vi "Intake Set.vi"() -> ()   [LabVIEW 2017]
uses:
  <vilib>/Rock Robotics/WPI/DriverStation/WPI_DriverStationRobotMode2.ctl
  Intake Control Type.ctl
  Intake Globals.vi
  Robot Global Data.vi
panel:
  out "error out 2":errorcluster
  out "error out":errorcluster
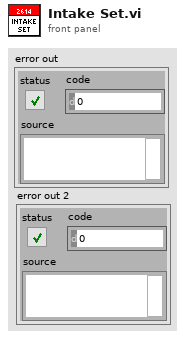
[diagram p1: front panel]
types:
  T1 = typedef "Intake Control Type.ctl" = enum16{"No Op", "In", "Out", "Test Mode", "Cube_In", "Cube_Out"}
  T2 = typedef "WPI_DriverStationRobotMode2.ctl" = enum16{"Autonomous Disabled", "Autonomous Enabled", "Teleop Disabled", "Teleop Enabled", "Disconnected", "Finish", "Test Disabled", "Test Enabled", "Emergency Stopped"}
  T3 = typedef "Intake Notifier.ctl" = cluster{"Intake Control Type":T1, "Step":i32, "In":bool, "Speed":dbl, "Out":bool, "Parameter 1":dbl, "Parameter 2":dbl, "Intake Notifier":refnum<notifier>, "Actuate Cube":bool, "Speed In":dbl, "Speed Out":dbl, "Load":bool, "Override":bool}
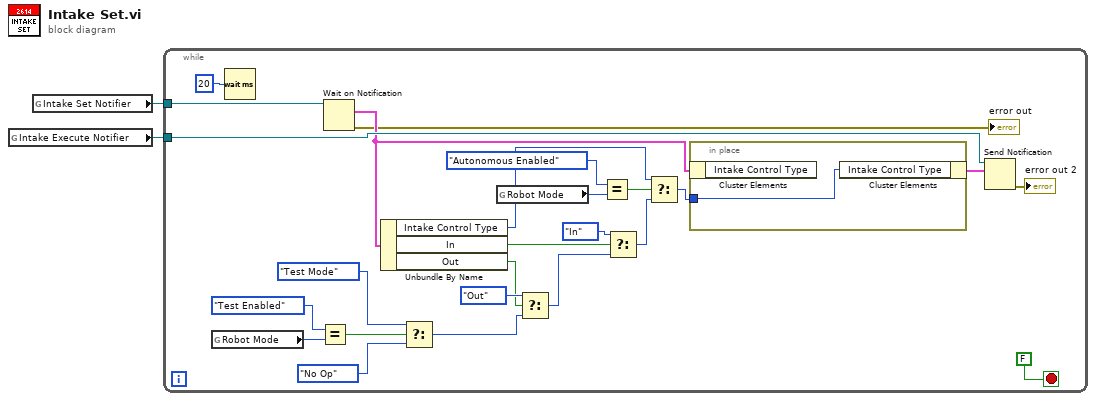
[diagram p0: block diagram]
diagram:
  n1 = global read "Intake Globals.vi" "Intake Execute Notifier"() -> (w1:refnum<notifier>)
  n2 = global read "Intake Globals.vi" "Intake Set Notifier"() -> (w2:refnum<notifier>)
  n3 = while {
    tunnel: w2 -> [w24]
    tunnel: w1 -> [w23]
    stop <- FALSE stop-if-true
    n4 = global read "Robot Global Data.vi" "Robot Mode"() -> (w10:T2)
    n5 = Wait (ms)(milliseconds to wait=u32 20) -> ()  [unwired: 1 out]
    n6 = Equal?(x=WPI_DriverStationRobotMode2."Test Enabled", y=w10) -> (x = y?=w8:bool)
    n7 = Wait on Notification(notifier=w24) -> (notification=w22:T3, error out=→"error out":errorcluster)  [unwired: 3 in, 2 out]
    n8 = Unbundle By Name(w22) -> ("Intake Control Type"=w18:T1, "In"=w14:bool, "Out"=w11:bool)
    n9 = Select(t=Intake_Control_Type."Test Mode", s=w8, f=Intake_Control_Type."No Op") -> (s? t:f=w6:T1)
    n10 = global read "Robot Global Data.vi" "Robot Mode"() -> (w20:T2)
    n11 = Select(t=Intake_Control_Type."Out", s=w11, f=w6) -> (s? t:f=w15:T1)
    n12 = Equal?(x=WPI_DriverStationRobotMode2."Autonomous Enabled", y=w20) -> (x = y?=w21:bool)
    n13 = Select(t=Intake_Control_Type."In", s=w14, f=w15) -> (s? t:f=w16:T1)
    n14 = Select(t=w18, s=w21, f=w16) -> (s? t:f=w17:T1)
    n15 = in-place {
      in-place-border: w17 -> [w28]
      n16 = in-place-cluster #1(w22) -> ()  [unwired: 1 out]
      n17 = in-place-cluster #1("Intake Control Type"=w28) -> (w25:T3)
    }
    n18 = Send Notification(notification=w25, notifier=w23) -> (error out=→"error out 2":errorcluster)  [unwired: 1 in, 1 out]
  }
